vi "Boolean Toggle.vi"(1 "Input":bool) -> (0 "Output":bool)   [LabVIEW 2013]
doc: "Changes a standard boolean input to a toggled boolean output."
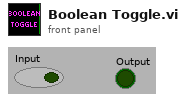
[diagram p1: front panel]
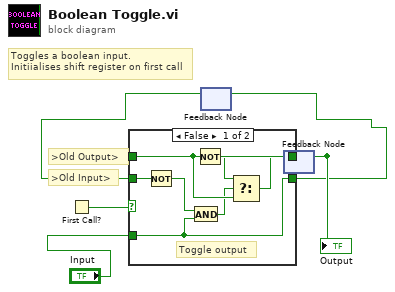
[diagram p0: block diagram]
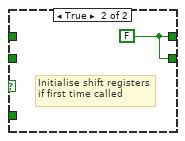
[diagram p2: hidden frame]
diagram:
  # ">Old Input>"
  # ">Old Output>"
  # "Toggles a boolean input.\nInitiialises shift register on first call"
  n1 = First Call?() -> (First Call?: T/F=w6:bool)
  n2 = feedback #1() -> (w1:bool)  [unwired: 1 in]
  n3 = feedback #2() -> (w3:bool)  [unwired: 1 in]
  "Output" <- w3
  n4 = case shown="False" w6 {
    tunnel: [w12 w14] -> w4
    tunnel: w3 -> [w11 _]
    tunnel: w1 -> [w7 _]
    tunnel: "Input" -> [w8 _]
    tunnel: [w8 w14] -> w2
    frame False {
      # "Toggle output"
      n5 = Not(x=w7) -> (.not. x?=w10:bool)
      n6 = And(x=w10, y=w8) -> (x .and. y?=w9:bool)
      n7 = Not(x=w11) -> (.not. x?=w13:bool)
      n8 = Select(t=w13, s=w9, f=w11) -> (s? t:f=w12:bool)
    }
    frame True {
      w14 = FALSE
      # "Initialise shift registers\nif first time called"
    }
  }
  n9 = feedback-in #1(w2) -> ()
  n10 = feedback-in #2(w4) -> ()
